vi "Read Card#.vi"(8 "error in (no error)":errorcluster, 11 "Power Meter Display in":refnum<class "Power Meter Display.lvclass">) -> (0 "error out":errorcluster, 2 "Card#":dbl, 3 "Power Meter Display out":refnum<class "Power Meter Display.lvclass">)   [LabVIEW 2012, in "Display Panel.lvlib" / "Power Meter Display.lvclass"]
uses:
  Power Meter Display.lvclass
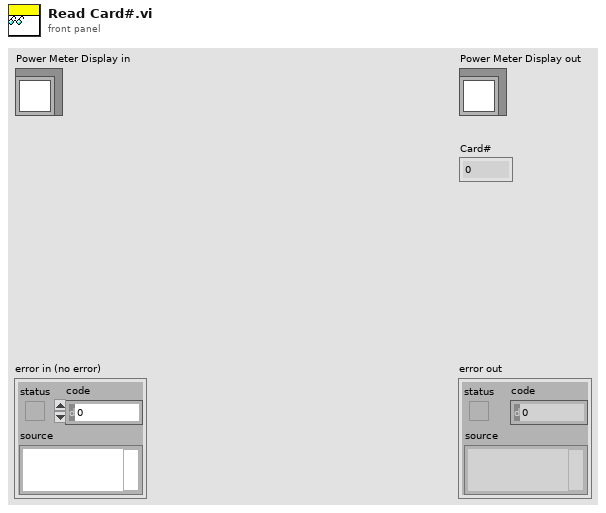
[diagram p1: front panel]
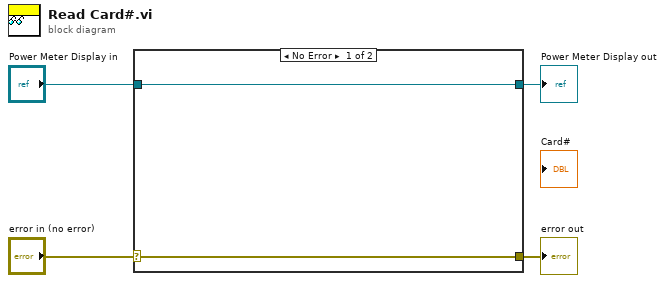
[diagram p0: block diagram]
diagram:
  n1 = case shown="No Error" "error in (no error)" {
    selector: "error in (no error)" -> [w6 w7]
    tunnel: [w6 w7] -> w3
    tunnel: [w5 w8] -> w1
    tunnel: "Power Meter Display in" -> [w5 w8]
    frame No Error {
    }
    frame Error {
    }
  }
  "error out" <- w3
  "Power Meter Display out" <- w1
